vi "通用报警记录浏览.vi"(11 "缓存数据路径":path=path "E:/Program Files (x86)/National Instruments/LabVIEW 2013/data/多点监测缓存数据文件-网络版/2016_10_23 00_23_16 #本机测试端口 #1.60 #1 #PC201410281258_8102.bin") -> ()   [LabVIEW 2017]
uses:
  <vilib>/Utility/miscctls.llb/LVAnnotationListTypeDef.ctl
  <vilib>/event_ctls.llb/eventvkey.ctl
  <vilib>/Utility/NIReport.llb/HTML Report Image Alignment.ctl
  <vilib>/Utility/NIReport.llb/Append Report Text (str wrap).vi
  <vilib>/Utility/NIReport.llb/Append Text Table to Report (wrap).vi
  <vilib>/printing/OpenHTMLReport.llb/Open HTML Report in Browser (Refnum).vi
  <vilib>/Utility/NIReport.llb/NI_report.lvclass
  <vilib>/Utility/NIReport.llb/NI_ReportGenerationCore.lvlib
panel:
  out "标题":string
  out "报警分析":i32(listbox)
  out "探测器信息":i32(listbox)
  out "数值":string
  in  "删除文件":bool
  in  "保存":bool
  out "路径显示":path=path "C:/Users/Administrator/Desktop/35点监测报警信息报表模板 - 副本.doc"
  in  "取消":bool
  in  "生成报表":bool
  in  "结论":string caption="结论（编辑）"
  out "实时曲线":cluster{"X":timestamp[], "Y":dbl[]}[](graph)
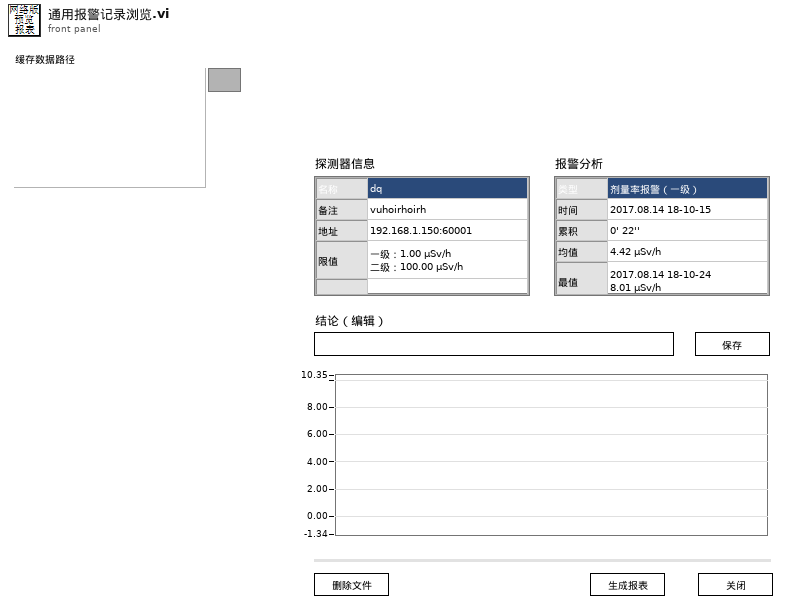
[diagram p1: front panel]
types:
  T1 = typedef "通用报警记录.ctl" = cluster{"探头状态":T2, "探头地址与信息":T3, "缓存绘图数据":T6, "平均值":dbl, "报警时长":cluster{"分":u16, "秒":u16}, "结论":string}
  T2 = typedef "探头状态.ctl" = enum16{"正常", "离线", "禁用", "一级报警", "二级报警", "累积报警"}
  T3 = typedef "探测器信息.ctl" = cluster{"网络地址":string, "名称":string, "备注":string, "累积剂量":dbl, "累积限值":dbl, "硬件剂量率限值":T4, "剂量率限值1":dbl, "剂量率限值2":dbl, "报警方式":T5}
  T4 = typedef "探头剂量率限值选择.ctl" = enum16{"一级限值", "二级限值"}
  T5 = typedef "报警方式选择.ctl" = enum16{"常报警", "自动静音", "手动静音"}
  T6 = typedef "时值缓存压缩模块.lvlib/缓存数据.ctl" = cluster{"时间":timestamp[], "数值":dbl[], "压缩等级数量":i32[], "最大值":cluster{"时间":timestamp, "数值":dbl}, "起始点":cluster{"时间":timestamp, "数值":dbl}, "容量限值":i32, "报警累积":dbl}
  T7 = typedef "LVAnnotationListTypeDef.ctl" = cluster{"Name":string, "Color":u32, "Style":u8, "Point Style":u8, "Name Visible":bool, "Allow Drag":bool, "Annotation Mode":u32, "Plot":i32, "Index":i32, "Position":cluster{"X":dbl, "Y":dbl}, "X Scale":u32, "Y Scale":u32, "Show Arrow":bool, "Lock Name":bool, "Plot Area":i32, "Label Offset":cluster{"X":dbl, "Y":dbl}}[]
  T8 = enum32{"Invalid", "Standard", "Closed", "Hidden", "Minimized", "Maximized"}
  T9 = typedef "eventvkey.ctl" = enum16{"ASCII", "Enter", "Return", "Shift", "Ctrl", "Alt", "Cmd", "Opt", "Caps", "NumLock", "Clear", "Break", "Up", "Down", "Left", "Right", "Insert", "Delete", "Home", "End", "PageUp", "PageDown", "Escape", "Help", "Pause", "ScrollLock", "F1", "F2", "F3", "F4", "F5", "F6", "F7", "F8", "F9", "F10", "F11", "F12", "F13", "F14", "F15", "F16", "F17", "F18", "F19", "F20", "F21", "F22", "F23", "F24", "Play", "VolumeUp", "VolumeDown", "Mute", "Two Byte Char"}
  T10 = enum16{"Standard Report", "HTML", "Word", "Excel"}
  T11 = typedef "NI_ReportGenerationCore.lvlib/HTML Report Image Alignment.ctl" = enum16{"(default)", "LEFT", "RIGHT", "TOP", "TEXTTOP", "MIDDLE", "ABSMIDDLE", "BASELINE", "BOTTOM", "ABSBOTTOM"}
  T12 = cluster{"Name":string, "Color":u32, "Style":u8, "Point Style":u8, "Name Visible":bool, "Allow Drag":bool, "Annotation Mode":u32, "Plot":i32, "Index":i32, "Position":cluster{"X":dbl, "Y":dbl}, "X Scale":u32, "Y Scale":u32, "Show Arrow":bool, "Lock Name":bool, "Plot Area":i32, "Label Offset":cluster{"X":dbl, "Y":dbl}}
  T13 = typedef "LVPoint32TypeDef.ctl" = cluster{"Horizontal":i32, "Vertical":i32}
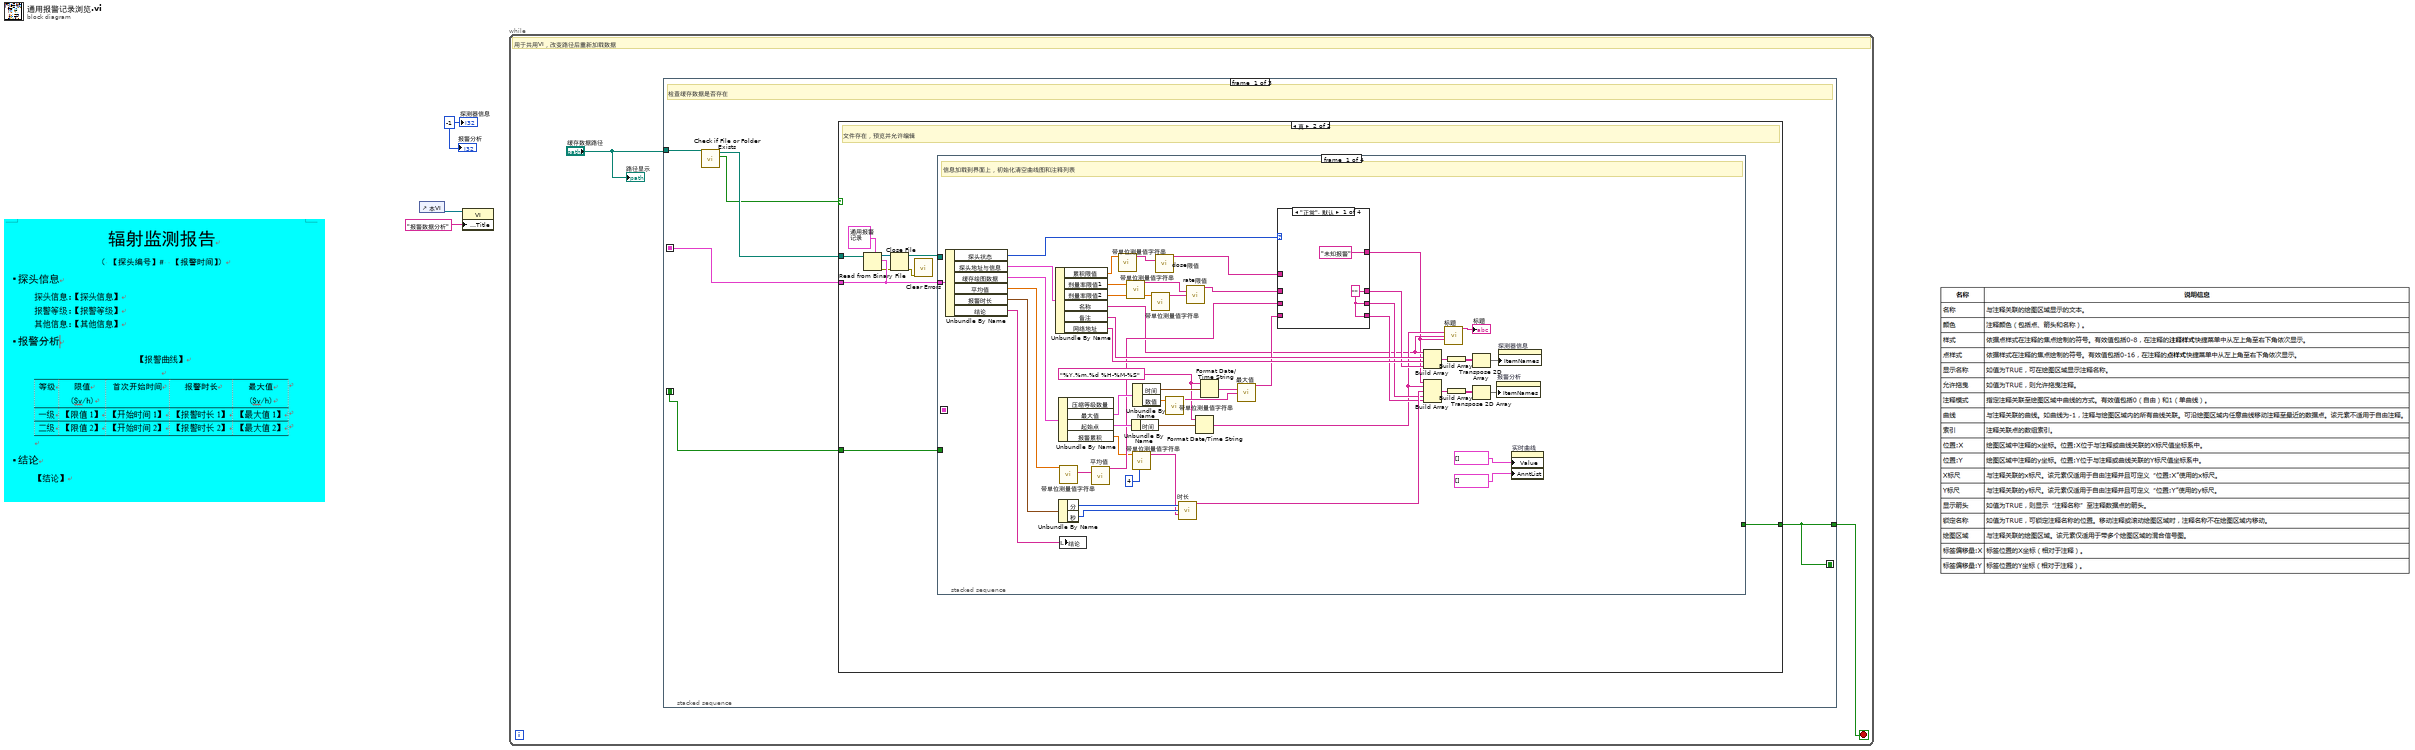
[diagram p0: block diagram]
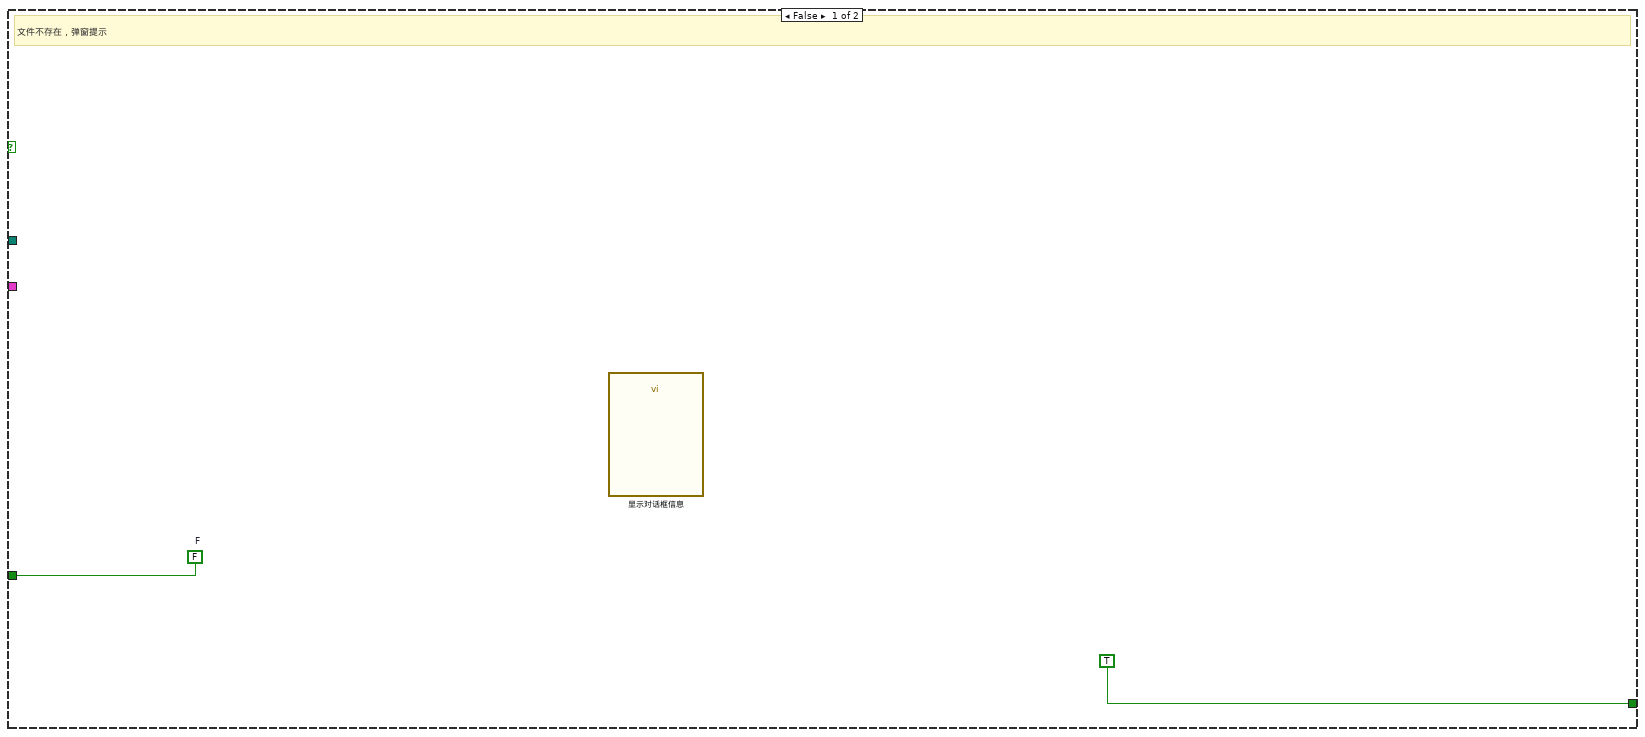
[diagram p2: hidden frame]
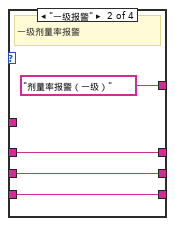
[diagram p3: hidden frame]
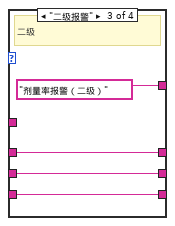
[diagram p4: hidden frame]
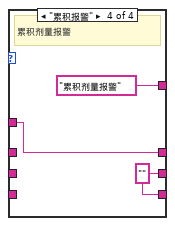
[diagram p5: hidden frame]
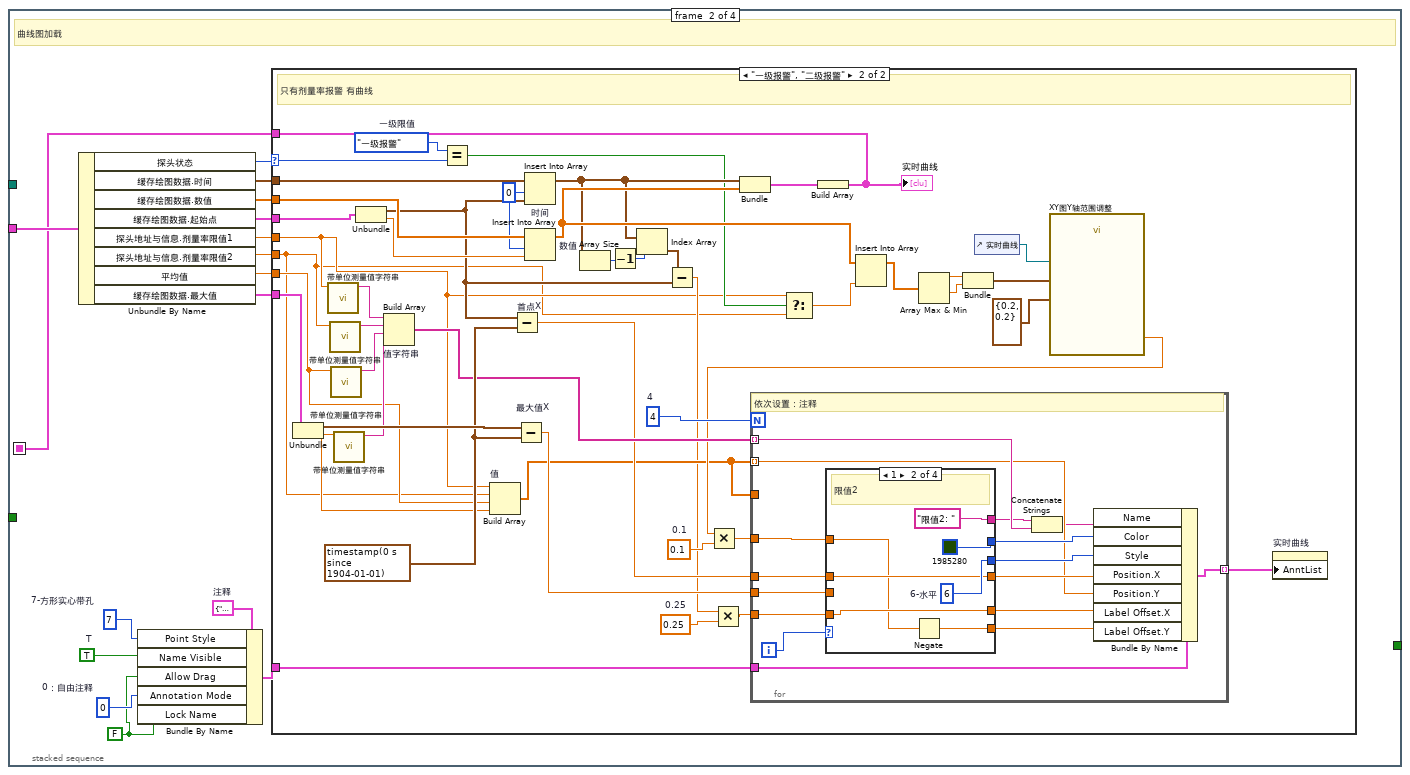
[diagram p6: hidden frame]
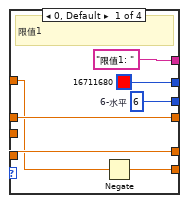
[diagram p8: hidden frame]
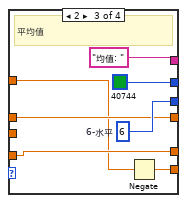
[diagram p9: hidden frame]
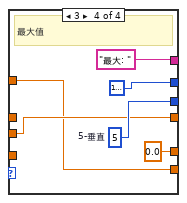
[diagram p10: hidden frame]
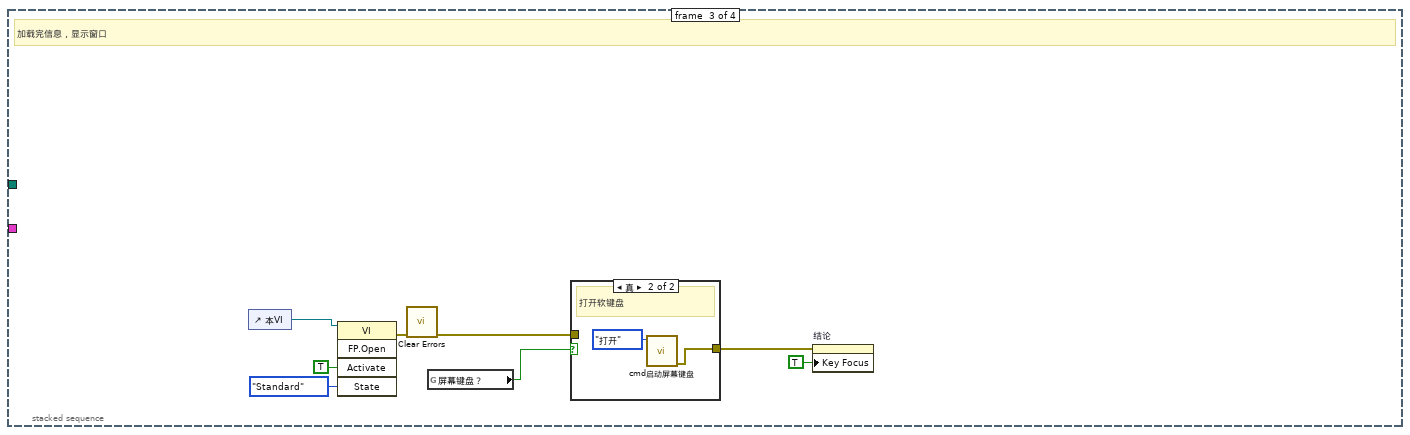
[diagram p11: hidden frame]
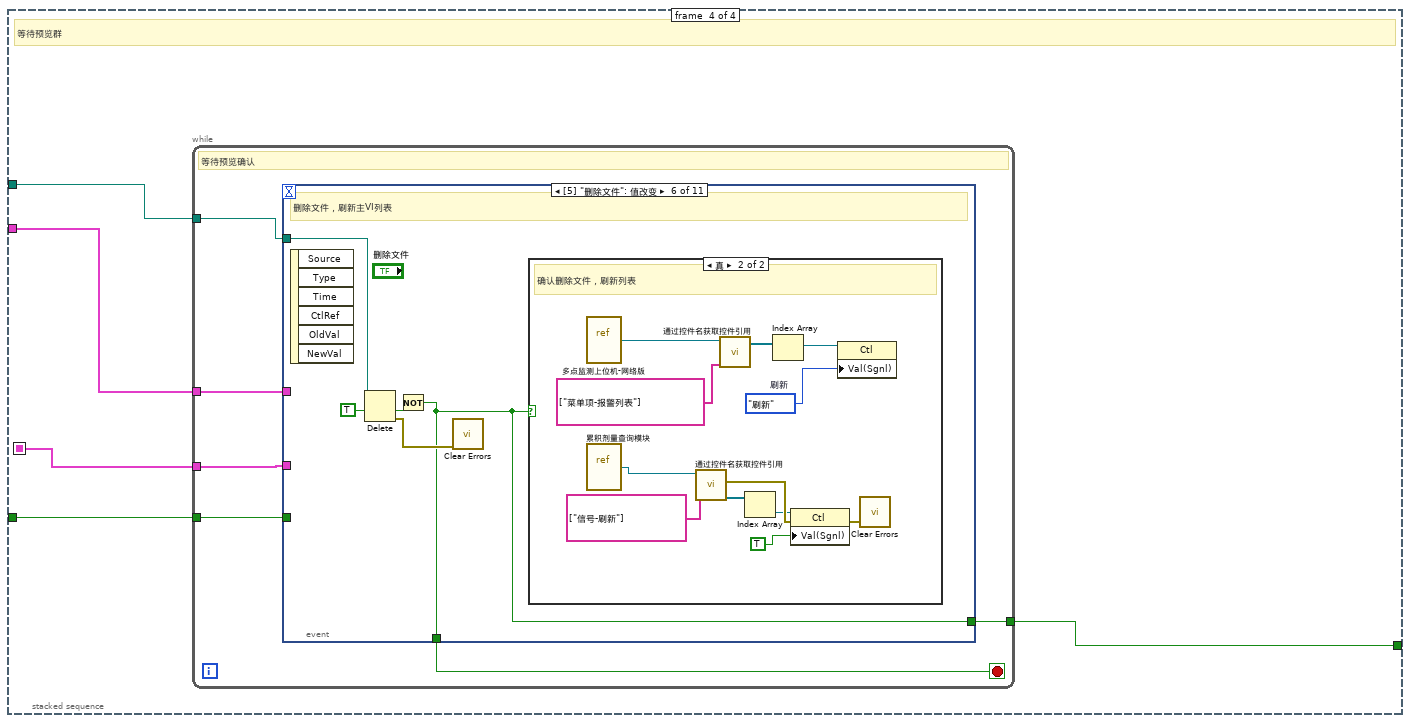
[diagram p13: hidden frame]
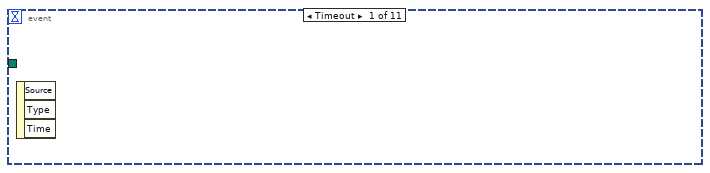
[diagram p14: hidden frame]
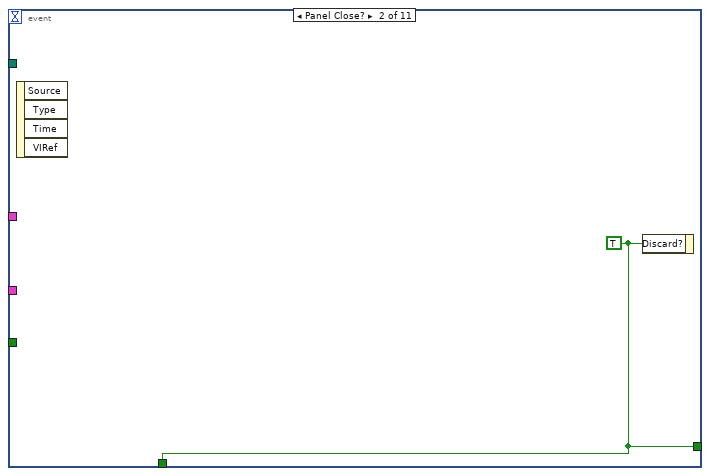
[diagram p15: hidden frame]
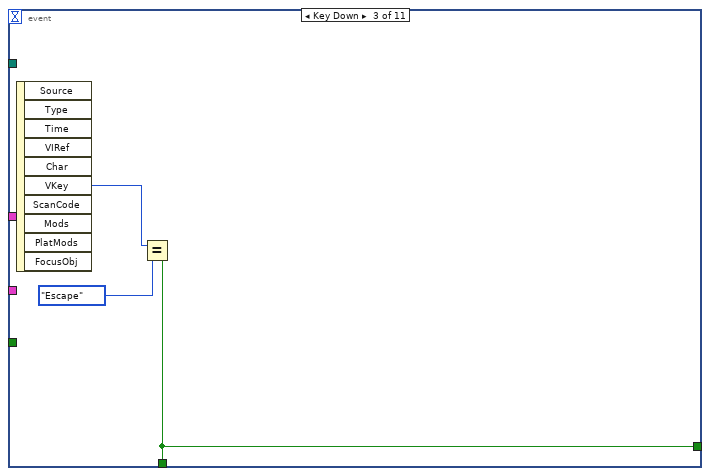
[diagram p16: hidden frame]
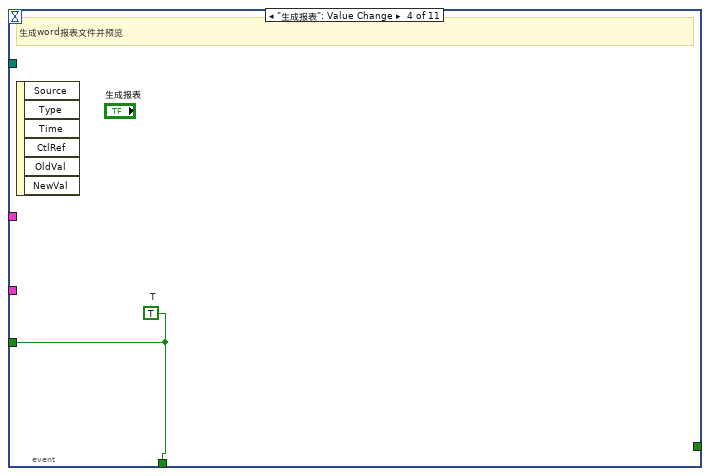
[diagram p17: hidden frame]
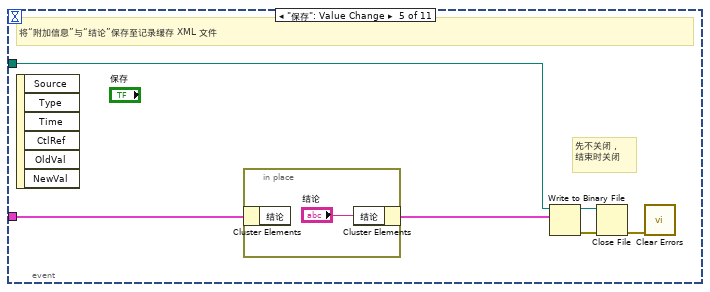
[diagram p18: hidden frame]
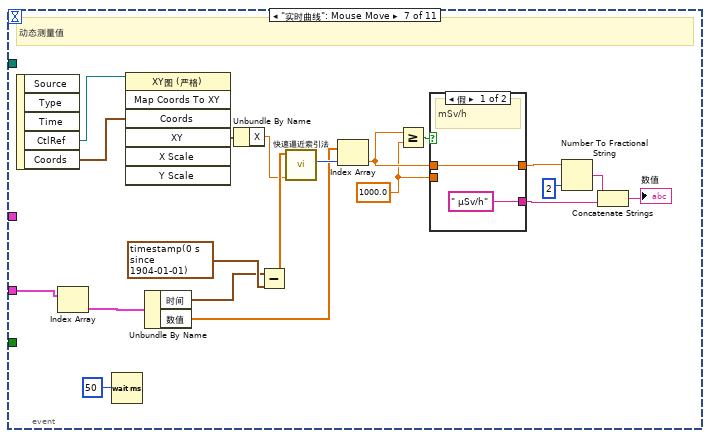
[diagram p20: hidden frame]
diagram:
  w1 = -1 ("探测器信息")
  n1 = control-ref of="本VI"() -> (w2:refnum<vi>)
  n2 = property class="VI"(reference=w2, "Front Panel.Title"="报警数据分析" ("前面板窗口:标题")) -> ()  [unwired: 1 in, 2 out]
  n3 = while {
    stop <- w4 stop-if-true
    # "用于共用VI，改变路径后重新加载数据"
    n4 = stacked-sequence {
      seq-local: [w11 _ _] -> [_ w275 _]
      seq-local: [w10 _ _] -> [_ _ w347]
      seq-local: [w6 _ _] -> [_ w273 _]
      tunnel: "缓存数据路径" -> [w9 w274 _]
      tunnel: [w10 _ _] -> w4
      frame #0 {
        # "检查缓存数据是否存在"
        n5 = call <vilib>:"Check if File or Folder Exists.vi"("path"=w9) -> ("file or folder exists?"=w7:bool, "dup path"=w8:path)  [unwired: 8 in, 1 out]
        n6 = case shown="真" w7 {
          tunnel: [_ w18] -> w6
          tunnel: [w13 w22] -> w11
          tunnel: w8 -> [_ w19]
          tunnel: [TRUE ("T") w21] -> w10
          frame False {
            w13 = FALSE  # F
            # "文件不存在，弹窗提示"
            n7 = call "显示对话框信息"() -> ()  [unwired: 10 in, 2 out]
          }
          frame True {
            # "文件存在，预览并允许编辑"
            n8 = Read from Binary File(5:T1 {"探头状态"=enum."正常", "探头地址与信息"={"网络地址"="", "名称"="", "备注"="", "累积剂量"=0.0, "累积限值"=0.0, "硬件剂量率限值"=enum."一级限值", "剂量率限值1"=0.0, "剂量率限值2"=0.0, "报警方式"=enum."常报警"}, "缓存绘图数据"={"时间"=[], "数值"=[], "压缩等级数量"=[], "最大值"={"时间"=timestamp(0 s since 1904-01-01), "数值"=0.0}, "起始点"={"时间"=timestamp(0 s since 1904-01-01), "数值"=0.0}, "容量限值"=0, "报警累积"=0.0}, "平均值"=0.0, "报警时长"={"分"=0, "秒"=0}, "结论"=""} ("报警记录"), 11:w19) -> (0:w16:errorcluster, 2:w18:T1, 3:w20:refnum<file>)  [unwired: 4 in, 1 out]
            n9 = Close File(refnum=w20, error in=w16) -> (path=w17:path, error out=w15:errorcluster)
            n10 = call <vilib>:"Clear Errors.vi"("error in (no error)"=w15) -> ()  [unwired: 5 in, 2 out]
            n11 = stacked-sequence {
              seq-local: [_ w87 _ _] -> [_ _ _ w201]
              tunnel: w18 -> [w71 w100 _ w204]
              tunnel: [_ _ _ w205] -> w22
              tunnel: w17 -> [_ _ _ w203]
              tunnel: [_ _ _ w202] -> w21
              frame #0 {
                w28 = "%Y.%m.%d %H-%M-%S" ("时间格式字符串(%c)")
                # "信息加载到界面上，初始化清空曲线图和注释列表"
                n12 = Unbundle By Name(w71) -> ("探头状态"=w64:T2, "探头地址与信息"=w69:T3, "缓存绘图数据"=w70:T6, "平均值"=w43:dbl, "报警时长"=w67:cluster{"分":u16, "秒":u16}, "结论"=w68:string)
                n13 = Unbundle By Name(w69) -> ("累积限值"=w61:dbl, "剂量率限值1"=w60:dbl, "剂量率限值2"=w59:dbl, "名称"=w31:string, "备注"=w63:string, "网络地址"=w62:string)
                n14 = Unbundle By Name(w70) -> ("最大值"=w46:cluster{"时间":timestamp, "数值":dbl}, "起始点"=w49:cluster{"时间":timestamp, "数值":dbl}, "报警累积"=w25:dbl)  [unwired: 1 out]
                n15 = Unbundle By Name(w67) -> ("分"=w66:u16, "秒"=w65:u16)
                n16 = local write "结论"(w68) -> ()
                n17 = call "带单位测量值字符串.vi"("测量值"=w43) -> ("结果"=w42:string)  [unwired: 10 in]
                n18 = call "平均值"("平均值"=w42) -> ("Result"=w39:string)  [unwired: 13 in, 1 out]
                n19 = call "带单位测量值字符串.vi"("测量值"=w61) -> ("结果"=w58:string)  [unwired: 10 in]
                n20 = call "带单位测量值字符串.vi"("测量值"=w60) -> ("结果"=w57:string)  [unwired: 10 in]
                n21 = Unbundle By Name(w49) -> ("时间"=w48:timestamp)
                n22 = call "带单位测量值字符串.vi"("精度(2)"=i16 4, "测量值"=w25) -> ("结果"=w24:string)  [unwired: 9 in]
                n23 = Unbundle By Name(w46) -> ("时间"=w45:timestamp, "数值"=w44:dbl)
                n24 = call "带单位测量值字符串.vi"("测量值"=w59) -> ("结果"=w56:string)  [unwired: 10 in]
                n25 = call "dose限值"("限值"=w58) -> ("Result"=w54:string)  [unwired: 13 in, 1 out]
                n26 = call "带单位测量值字符串.vi"("测量值"=w44) -> ("结果"=w40:string)  [unwired: 10 in]
                n27 = call "时长"("分"=w66, "秒"=w65, "累积"=w24) -> ("Result"=w47:string)  [unwired: 11 in, 1 out]
                n28 = call "rate限值"("限值1"=w57, "限值2"=w56) -> ("Result"=w55:string)  [unwired: 12 in, 1 out]
                n29 = Format Date/Time String(time format string (%c)=w28, seconds (now)=w48) -> (date/time string=w32:string)  [unwired: 1 in]
                n30 = Format Date/Time String(time format string (%c)=w28, seconds (now)=w45) -> (date/time string=w41:string)  [unwired: 1 in]
                n31 = call "最大值"("时间"=w41, "最大值"=w40) -> ("Result"=w38:string)  [unwired: 12 in, 1 out]
                n32 = case shown="\"正常\", 默认" w64 {
                  tunnel: ["未知报警" ("字符串") "剂量率报警（一级）" ("字符串") "剂量率报警（二级）" ("字符串") "累积剂量报警" ("字符串")] -> w30
                  tunnel: w55 -> [_ w76 w80 _]
                  tunnel: w54 -> [_ _ _ w83]
                  tunnel: [w72 w76 w80 w83] -> w53
                  tunnel: w39 -> [_ w75 w79 _]
                  tunnel: w38 -> [_ w74 w78 _]
                  tunnel: [w72 w75 w79 w82] -> w37
                  tunnel: [w72 w74 w78 w82] -> w36
                  frame "正常", Default {
                    w72 = "" ("Result")
                  }
                  frame "一级报警" {
                    # "一级剂量率报警"
                  }
                  frame "二级报警" {
                    # "二级"
                  }
                  frame "累积报警" {
                    w82 = "" ("Result")
                    # "累积剂量报警"
                  }
                }
                n33 = Build Array(w31, w63, w62, w53) -> (w52:string[])
                n34 = Build Array(w30, w32, w47, w37, w36) -> (w34:string[])
                n35 = call "标题"("时间"=w32, "名称"=w31, "类型"=w30) -> ("Result"=→"标题":string)  [unwired: 11 in, 1 out]
                n36 = Build Array(w52) -> (w51:string[][])
                n37 = Build Array(w34) -> (w35:string[][])
                n38 = Transpose 2D Array(2D array=w51) -> (transposed array=w50:string[][])
                n39 = Transpose 2D Array(2D array=w35) -> (transposed array=w33:string[][])
                n40 = property on="报警分析" class="MCListbox (严格)"("ItemNames"=w33) -> ()  [unwired: 2 in, 2 out]
                n41 = property on="探测器信息" class="MCListbox (严格)"("ItemNames"=w50) -> ()  [unwired: 2 in, 2 out]
                n42 = property on="实时曲线" class="XY图 (严格)"("Value"=cluster{"X":timestamp[], "Y":dbl[]}[] [] ("实时曲线"), "AnntList"=T7 [] ("注释列表")) -> ()  [unwired: 2 in, 2 out]
              }
              frame #1 {
                w85 = FALSE ("Lock Name")
                w89 = u32 0  # 0：自由注释
                w86 = TRUE  # T
                w90 = 7  # 7-方形实心带孔
                w91 = T12 {"Name"="", "Color"=0, "Style"=0, "Point Style"=0, "Name Visible"=FALSE, "Allow Drag"=FALSE, "Annotation Mode"=0, "Plot"=0, "Index"=0, "Position"={"X"=0.0, "Y"=0.0}, "X Scale"=0, "Y Scale"=0, "Show Arrow"=FALSE, "Lock Name"=FALSE, "Plot Area"=0, "Label Offset"={"X"=0.0, "Y"=0.0}}  # 注释
                # "曲线图加载"
                n43 = Unbundle By Name(w100) -> ("探头状态"=w92:T2, "缓存绘图数据.时间"=w97:timestamp[], "缓存绘图数据.数值"=w98:dbl[], "缓存绘图数据.起始点"=w99:cluster{"时间":timestamp, "数值":dbl}, "探头地址与信息.剂量率限值1"=w96:dbl, "探头地址与信息.剂量率限值2"=w95:dbl, "平均值"=w94:dbl, "缓存绘图数据.最大值"=w93:cluster{"时间":timestamp, "数值":dbl})
                n44 = Bundle By Name(cluster=w91, "Point Style"=w90, "Name Visible"=w86, "Allow Drag"=w85, "Annotation Mode"=w89, "Lock Name"=w85) -> (w88:T12)
                n45 = case shown="\"一级报警\", \"二级报警\"" w92 {
                  selector: w92 -> [_ w106]
                  tunnel: w99 -> [_ w147]
                  tunnel: w98 -> [_ w145]
                  tunnel: w97 -> [_ w143]
                  tunnel: w96 -> [_ w103]
                  tunnel: w95 -> [_ w102]
                  tunnel: w94 -> [_ w132]
                  tunnel: w93 -> [_ w142]
                  tunnel: w88 -> [_ w138]
                  tunnel: [_ w127] -> w87
                  frame "正常", Default {
                  }
                  frame "一级报警", "二级报警" {
                    w105 = 探头状态."一级报警"  # 一级限值
                    w116 = 0.25  # 0.25
                    w118 = 0.1  # 0.1
                    w126 = 0 ("索引")
                    w139 = 4  # 4
                    w140 = timestamp(0 s since 1904-01-01)
                    # "只有剂量率报警 有曲线"
                    n46 = Unbundle(w142) -> ("时间"=w141:timestamp, "数值"=w133:dbl)
                    n47 = call "带单位测量值字符串.vi"("测量值"=w103) -> ("结果"=w137:string)  [unwired: 10 in]
                    n48 = call "带单位测量值字符串.vi"("测量值"=w102) -> ("结果"=w136:string)  [unwired: 10 in]
                    n49 = call "带单位测量值字符串.vi"("测量值"=w132) -> ("结果"=w135:string)  [unwired: 10 in]
                    n50 = call "带单位测量值字符串.vi"("测量值"=w133) -> ("结果"=w134:string)  [unwired: 10 in]
                    n51 = Unbundle(w147) -> ("时间"=w109:timestamp, "数值"=w146:dbl)
                    n52 = Build Array "值字符串"(w137, w136, w135, w134) -> (w131:string[])
                    n53 = Equal?(x=w105, y=w106) -> (x = y?=w104:bool)
                    n54 = Build Array "值"(w103, w102, w132, w133) -> (w114:dbl[])
                    n55 = Subtract "首点X"(x=w109, y=w140) -> (x-y=w130:dbl)
                    n56 = Subtract "最大值X"(x=w141, y=w140) -> (x-y=w129:dbl)
                    n57 = Insert Into Array "时间"(array=w143, index=w126, new element=w109) -> (w112:timestamp[])
                    n58 = Insert Into Array "数值"(array=w145, index=w126, new element=w146) -> (w125:dbl[])
                    n59 = Array Size(array=w112) -> (size(s)=w113:i32)
                    n60 = Decrement(x=w113) -> (x-1=w111:i32)
                    n61 = Index Array(array=w112, index=w111) -> (element=w110:timestamp)
                    n62 = Subtract(x=w110, y=w109) -> (x-y=w108:dbl)
                    n63 = Multiply(x=w108, y=w116) -> (x*y=w115:dbl)
                    n64 = Bundle("时间"=w112, "数值"=w125) -> (w144:cluster{"时间":timestamp[], "数值":dbl[]})  [unwired: 1 in]
                    n65 = Select(t=w103, s=w104, f=w102) -> (s? t:f=w101:dbl)
                    n66 = Build Array(w144) -> (w127:cluster{"时间":timestamp[], "数值":dbl[]}[])
                    "实时曲线" <- w127
                    n67 = Insert Into Array(array=w125, new element=w101) -> (w107:dbl[])  [unwired: 1 in]
                    n68 = Array Max & Min(array=w107) -> (max value=w124:dbl, min value=w123:dbl)  [unwired: 2 out]
                    n69 = Bundle(w124, w123) -> (w122:cluster{dbl, dbl})  [unwired: 1 in]
                    n70 = control-ref of="实时曲线"() -> (w120:refnum<vi>)
                    n71 = call "XY图Y轴范围调整.vi"("留白比例"=cluster{"顶白比例":dbl, "底白比例":dbl} {"顶白比例"=0.2, "底白比例"=0.2}, "最值"=w122, "XY图引用"=w120) -> ("Y轴全长"=w117:dbl)  [unwired: 6 in, 2 out]
                    n72 = Multiply(x=w117, y=w118) -> (x*y=w119:dbl)
                    n73 = for {
                      N: w139 -> [_]
                      tunnel: w138 -> [w162]
                      tunnel: w131 -> [w161] mode=indexing
                      tunnel: w130 -> [w158]
                      tunnel: w129 -> [w157]
                      tunnel: w114 -> [w155] mode=indexing
                      tunnel: w115 -> [w154]
                      tunnel: [w152] -> w128 mode=indexing
                      tunnel: w119 -> [w149]
                      tunnel: w114 -> [_]
                      i -> [w163]
                      # "依次设置：注释"
                      n74 = case shown="1" w163 {
                        tunnel: [u32 16711680 u32 1985280 u32 40744 u32 16777224] -> w160
                        tunnel: [w169 w176 w183 w189] -> w159
                        tunnel: w158 -> [w168 w175 w182 _]
                        tunnel: w157 -> [_ _ _ w186]
                        tunnel: [w168 w175 w182 w186] -> w156
                        tunnel: w154 -> [w167 w174 w181 _]
                        tunnel: [w167 w174 w181 0.0] -> w153
                        tunnel: ["限值1: " "限值2: " "均值: " "最大: "] -> w150
                        tunnel: w149 -> [w165 w172 w179 w185]
                        tunnel: [w164 w171 w178 w185] -> w148
                        frame 0, Default {
                          w169 = u8 6  # 6-水平
                          # "限值1"
                          n75 = Negate(x=w165) -> (-x=w164:dbl)
                        }
                        frame 1 {
                          w176 = u8 6  # 6-水平
                          # "限值2"
                          n76 = Negate(x=w172) -> (-x=w171:dbl)
                        }
                        frame 2 {
                          w183 = u8 6  # 6-水平
                          # "平均值"
                          n77 = Negate(x=w179) -> (-x=w178:dbl)
                        }
                        frame 3 {
                          w189 = u8 5  # 5-垂直
                          # "最大值"
                        }
                      }
                      n78 = Concatenate Strings(w150, w161) -> (w151:string)
                      n79 = Bundle By Name(cluster=w162, "Name"=w151, "Color"=w160, "Style"=w159, "Position.X"=w156, "Position.Y"=w155, "Label Offset.X"=w153, "Label Offset.Y"=w148) -> (w152:T12)
                    }
                    n80 = property on="实时曲线" class="XY图 (严格)"("AnntList"=w128) -> ()  [unwired: 2 in, 2 out]
                  }
                }
              }
              frame #2 {
                # "加载完信息，显示窗口"
                n81 = control-ref of="本VI"() -> (w198:refnum<vi>)
                n82 = invoke class="VI" method="FP.Open"(reference=w198, "Activate"=TRUE ("激活？"), "State"=T8."Standard" ("状态")) -> (error out=w195:errorcluster)  [unwired: 2 in, 4 out]
                n83 = call <vilib>:"Clear Errors.vi"("error in (no error)"=w195) -> ("error out"=w192:errorcluster)  [unwired: 5 in, 1 out]
                n84 = global read "全局变量-35点监测.vi" "屏幕键盘？"() -> (w191:bool)
                n85 = case shown="真" w191 {
                  tunnel: [_ w199] -> w193
                  tunnel: w192 -> [_ _]
                  frame False {
                  }
                  frame True {
                    # "打开软键盘"
                    n86 = call "cmd启动屏幕键盘.vi"("软键盘开关"=enum16{"关闭", "打开"}."打开") -> ("error out"=w199:errorcluster)  [unwired: 9 in, 1 out]
                  }
                }
                n87 = property on="结论" class="Str"(error in=w193, "Key Focus"=TRUE ("键选中")) -> ()  [unwired: 1 in, 2 out]
              }
              frame #3 {
                # "等待预览群"
                n88 = while {
                  tunnel: [w210] -> w205
                  tunnel: w204 -> [w209]
                  tunnel: w203 -> [w208]
                  tunnel: [w207] -> w202
                  tunnel: w201 -> [w206]
                  stop <- w211 stop-if-true
                  # "等待预览确认"
                  n89 = event shown="[5] \"删除文件\": 值改变" {
                    selector: _ -> [_ _ _ _ _ _ _ _ _ _ _]
                    dyn-events: _ -> [_ _ _ _ _ _ _ _ _ _ _]
                    timeout: _ -> [_ _ _ _ _ _ _ _ _ _ _]
                    tunnel: [_ w212 w213 w216 _ w224 _ _ _ TRUE ("T") w271] -> w211
                    tunnel: [_ _ _ w216 _ _ _ _ _ _ w272] -> w210
                    tunnel: w209 -> [_ _ _ _ w222 _ _ _ _ _ _]
                    tunnel: w208 -> [_ _ _ _ w221 w227 _ _ _ _ _]
                    tunnel: [_ w212 w213 _ _ w224 _ _ _ FALSE ("T") w271] -> w207
                    tunnel: w206 -> [_ _ _ _ _ _ w241 _ _ _ _]
                    event Timeout {
                      n90 = event-data() -> ()  [unwired: 1 in, 3 out]
                    }
                    event Panel Close? {
                      w212 = TRUE ("放弃？")
                      n91 = event-data() -> ()  [unwired: 1 in, 4 out]
                      n92 = event-data("Discard?"=w212) -> ()  [unwired: 1 in, 1 out]
                    }
                    event Key Down {
                      n93 = event-data() -> ("VKey"=w215:T9)  [unwired: 1 in, 9 out]
                      n94 = Equal?(x=w215, y=eventvkey."Escape") -> (x = y?=w213:bool)
                    }
                    event "生成报表": Value Change {
                      w216 = TRUE  # T
                      # "生成word报表文件并预览"
                      n95 = event-data() -> ()  [unwired: 1 in, 6 out]
                    }
                    event "保存": Value Change {
                      # "先不关闭，\n结束时关闭"
                      # "将“附加信息”与“结论”保存至记录缓存 XML 文件"
                      n96 = event-data() -> ()  [unwired: 1 in, 6 out]
                      n97 = in-place {
                        n98 = in-place-cluster #1(w222) -> ()  [unwired: 1 out]
                        n99 = in-place-cluster #1("结论"="结论") -> (w220:T1)
                      }
                      n100 = Write to Binary File(file (use dialog)=w221, data=w220) -> (refnum out=w217:refnum<file>, error out=w219:errorcluster)  [unwired: 4 in, 1 out]
                      n101 = Close File(refnum=w217, error in=w219) -> (error out=w218:errorcluster)  [unwired: 1 out]
                      n102 = call <vilib>:"Clear Errors.vi"("error in (no error)"=w218) -> ()  [unwired: 5 in, 2 out]
                    }
                    event "删除文件": Value Change {
                      # "删除文件，刷新主VI列表"
                      n103 = event-data() -> ()  [unwired: 1 in, 6 out]
                      n104 = Delete(path (use dialog)=w227, confirm (F)=TRUE ("确认(F)")) -> (cancelled=w225:bool, error out=w228:errorcluster)  [unwired: 3 in, 1 out]
                      n105 = Not(x=w225) -> (.not. x?=w224:bool)
                      n106 = call <vilib>:"Clear Errors.vi"("error in (no error)"=w228) -> ()  [unwired: 5 in, 2 out]
                      n107 = case shown="真" w224 {
                        frame False {
                          # "取消删除"
                        }
                        frame True {
                          w236 = enum16{"刷新", "预览并生成报表", "删除记录", "复制选中项至剪贴板"}."刷新"  # 刷新
                          # "确认删除文件，刷新列表"
                          n108 = vi-ref "多点监测上位机-网络版.vi"() -> (w240:refnum<vi>)
                          n109 = vi-ref "累积剂量查询模块.vi"() -> (w230:refnum<vi>)
                          n110 = call "通过控件名获取控件引用.vi"("控件名数组"=string[] ["信号-刷新"], "VI引用"=w230) -> ("控件引用输出"=w231:refnum<vi>[], "错误输出"=w234:errorcluster)  [unwired: 7 in, 1 out]
                          n111 = call "通过控件名获取控件引用.vi"("控件名数组"=string[] ["菜单项-报警列表"], "VI引用"=w240) -> ("控件引用输出"=w238:refnum<vi>[])  [unwired: 7 in, 2 out]
                          n112 = Index Array(array=w231) -> (element=w232:refnum<vi>)  [unwired: 1 in]
                          n113 = Index Array(array=w238) -> (element=w237:refnum<vi>)  [unwired: 1 in]
                          n114 = property class="Ctl"(reference=w232, error in=w234, "Val(Sgnl)"=TRUE) -> (error out=w235:errorcluster)  [unwired: 1 out]
                          n115 = property class="Ctl"(reference=w237, "Val(Sgnl)"=w236) -> ()  [unwired: 1 in, 2 out]
                          n116 = call <vilib>:"Clear Errors.vi"("error in (no error)"=w235) -> ()  [unwired: 5 in, 2 out]
                        }
                      }
                    }
                    event "实时曲线": Mouse Move {
                      w248 = 1000.0 ("y")
                      # "动态测量值"
                      n117 = event-data() -> ("CtlRef"=w243:refnum<vi>, "Coords"=w244:T13)  [unwired: 1 in, 3 out]
                      n118 = Index Array(array=w241) -> (element=w242:cluster{"时间":timestamp[], "数值":dbl[]})  [unwired: 1 in]
                      n119 = Wait (ms)(milliseconds to wait=u32 50 ("等待时间（毫秒）")) -> ()  [unwired: 1 out]
                      n120 = invoke on="调用节点" class="XY图 (严格)" method="Map Coords To XY"(reference=w243, "Coords"=w244) -> ("XY"=w246:cluster{"X":dbl, "Y":dbl})  [unwired: 5 in, 6 out]
                      n121 = Unbundle By Name(w242) -> ("时间"=w255:timestamp[], "数值"=w258:dbl[])
                      n122 = Unbundle By Name(w246) -> ("X"=w254:dbl)
                      n123 = Subtract(x=w255, y=timestamp(0 s since 1904-01-01)) -> (x-y=w257:dbl[])
                      n124 = call "快速逼近索引法.vi"("数值"=w254, "数组"=w257) -> ("最近索引"=w259:i32)  [unwired: 9 in]
                      n125 = Index Array(array=w258, index=w259) -> (element=w260:dbl)
                      n126 = Greater Or Equal?(x=w260, y=w248) -> (x >= y?=w247:bool)
                      n127 = case shown="假" w247 {
                        tunnel: w260 -> [w262 w266]
                        tunnel: w248 -> [_ w265]
                        tunnel: [w262 w264] -> w250
                        tunnel: [" μSv/h" " mSv/h"] -> w252
                        frame False {
                          # "mSv/h"
                        }
                        frame True {
                          # "uSv/h"
                          n128 = Divide(x=w266, y=w265) -> (x/y=w264:dbl)
                        }
                      }
                      n129 = Number To Fractional String(number=w250, precision (6)=i16 2 ("精度(6)")) -> (F-format string=w251:string)  [unwired: 2 in]
                      n130 = Concatenate Strings(w251, w252) -> (→"数值":string)
                    }
                    event "实时曲线": Mouse Enter {
                      # "显示 动态测量值"
                      n131 = event-data() -> ()  [unwired: 1 in, 4 out]
                      n132 = property on="数值" class="Str"("Visible"=TRUE ("可见")) -> ()  [unwired: 2 in, 2 out]
                    }
                    event "实时曲线": Mouse Leave {
                      # "隐藏 动态测量值"
                      n133 = event-data() -> ()  [unwired: 1 in, 4 out]
                      n134 = property on="数值" class="Str"("Visible"=FALSE ("可见")) -> ()  [unwired: 2 in, 2 out]
                    }
                    event "缓存数据路径": Value Change {
                      # "重新加载与分析数据，结束当前循环"
                      n135 = event-data() -> ()  [unwired: 1 in, 6 out]
                    }
                    event "取消": Value Change {
                      w272 = FALSE  # F
                      w271 = TRUE  # T
                      # "取消生成"
                      n136 = event-data() -> ()  [unwired: 1 in, 6 out]
                    }
                  }
                }
              }
            }
          }
        }
      }
      frame #1 {
        # "是否生成报表"
        n137 = case shown="真" w275 {
          tunnel: w274 -> [_ _]
          tunnel: w273 -> [_ w337]
          frame False {
            # "缓存数据不存在，或点击“取消”"
          }
          frame True {
            w290 = 1.75
            w324 = enum16{"H1", "H2", "H3", "H4", "H5", "H6", "H7"}."H3"  # H1
            w315 = FALSE  # F
            w302 = TRUE  # T
            w332 = TRUE  # T
            w298 = FALSE  # F
            # "缓存数据存在，并点击“生成报表”，生成 HTML 报表"
            n138 = Unbundle By Name(w337) -> ("探头状态"=w310:T2)
            n139 = local read "标题"() -> (w326:string)
            n140 = call <vilib>:"New Report.vi"("report type"=T10."HTML") -> ("report out"=w328:refnum<class "NI_report.lvclass">, "error out"=w327:errorcluster)  [unwired: 13 in]
            n141 = call-dynamic "Set Report Header Text.vi"("report in"=w328, "center header text"=w326, "error in (no error)"=w327, "HTML header size"=w324, "header placement"=enum16{"Top of Document", "Append to Body"}."Append to Body") -> ("report out"=w320:refnum<class "NI_report.lvclass">, "error out"=w319:errorcluster)  [unwired: 9 in]
            n142 = property on="探测器信息" class="MCListbox (严格)"() -> ("RowHdrs[]"=w314:string[], "ItemNames"=w313:string[][])  [unwired: 2 in, 2 out]
            n143 = call-poly <vilib>:"Append Report Text.vi"("report in"=w320, "text"="\n一、探测器信息\n", "append on new line? (F)"=w302, "error in (no error)"=w319) -> ("report out"=w282:refnum<class "NI_report.lvclass">, "error out"=w283:errorcluster)  [unwired: 8 in, 2 out]
            n144 = call-dynamic "New Report Line.vi"("report in"=w282, "error in (no error)"=w283) -> ("report out"=w281:refnum<class "NI_report.lvclass">, "error out"=w280:errorcluster)  [unwired: 12 in]
            n145 = call-poly <vilib>:"Append Table to Report.vi"("report in"=w281, "column width (1)"=w290, "row headers"=w314, "text data"=w313, "error in (no error)"=w280, "show grid lines (YES)"=w315) -> ("report out"=w284:refnum<class "NI_report.lvclass">, "error out"=w285:errorcluster)  [unwired: 6 in, 2 out]
            n146 = property on="报警分析" class="MCListbox (严格)"() -> ("RowHdrs[]"=w312:string[], "ItemNames"=w311:string[][])  [unwired: 2 in, 2 out]
            n147 = call-poly <vilib>:"Append Report Text.vi"("report in"=w284, "text"="二、报警分析\n", "append on new line? (F)"=w302, "error in (no error)"=w285) -> ("report out"=w289:refnum<class "NI_report.lvclass">, "error out"=w287:errorcluster)  [unwired: 8 in, 2 out]
            n148 = call-dynamic "New Report Line.vi"("report in"=w289, "error in (no error)"=w287) -> ("report out"=w288:refnum<class "NI_report.lvclass">, "error out"=w286:errorcluster)  [unwired: 12 in]
            n149 = call-poly <vilib>:"Append Table to Report.vi"("report in"=w288, "column width (1)"=w290, "row headers"=w312, "text data"=w311, "error in (no error)"=w286, "show grid lines (YES)"=w315) -> ("report out"=w278:refnum<class "NI_report.lvclass">, "error out"=w279:errorcluster)  [unwired: 6 in, 2 out]
            n150 = call-dynamic "New Report Line.vi"("report in"=w278, "error in (no error)"=w279) -> ("report out"=w277:refnum<class "NI_report.lvclass">, "error out"=w276:errorcluster)  [unwired: 12 in]
            n151 = case shown="\"一级报警\", \"二级报警\"" w310 {
              tunnel: w277 -> [w339 w346]
              tunnel: w276 -> [w338 w345]
              tunnel: [w338 w341] -> w309
              tunnel: [w339 w340] -> w308
              frame "禁用", Default {
                # "累积剂量报警没有曲线图"
              }
              frame "一级报警", "二级报警" {
                # "剂量率报警有曲线图"
                n152 = control-ref of="实时曲线"() -> (w344:refnum<vi>)
                n153 = call-dynamic "Append Control Image to Report.vi"("report in"=w346, "alignment (default)"=HTML_Report_Image_Alignment."MIDDLE", "image file type (.jpg)"=enum16{".jpg", ".png"}.".png", "ctrl reference"=w344, "error in (no error)"=w345) -> ("report out"=w340:refnum<class "NI_report.lvclass">, "error out"=w341:errorcluster)  [unwired: 7 in, 2 out]
              }
            }
            n154 = call "路径查找创建-报警记录清单-网络版.vi"() -> ("报表文件夹"=w331:path)  [unwired: 2 in, 13 out]
            n155 = call-poly <vilib>:"Append Report Text.vi"("report in"=w308, "text"="\n三、结论\n", "append on new line? (F)"=w302, "error in (no error)"=w309) -> ("report out"=w317:refnum<class "NI_report.lvclass">, "error out"=w316:errorcluster)  [unwired: 8 in, 2 out]
            n156 = local read "结论"() -> (w318:string)
            n157 = call-poly <vilib>:"Append Report Text.vi"("report in"=w317, "text"=w318, "append on new line? (F)"=w302, "error in (no error)"=w316) -> ("report out"=w305:refnum<class "NI_report.lvclass">, "error out"=w306:errorcluster)  [unwired: 8 in, 2 out]
            n158 = call-dynamic "New Report Line.vi"("report in"=w305, "number of lines (1)"=2, "error in (no error)"=w306) -> ("report out"=w304:refnum<class "NI_report.lvclass">, "error out"=w303:errorcluster)  [unwired: 11 in]
            n159 = Concatenate Strings(w326, ".html" ("字符串")) -> (w296:string)
            n160 = call-dynamic "Append Horizontal Line to Report.vi"("report in"=w304, "error in (no error)"=w303) -> ("report out"=w301:refnum<class "NI_report.lvclass">, "error out"=w299:errorcluster)  [unwired: 12 in]
            n161 = call-poly <vilib>:"Append Report Text.vi"("report in"=w301, "text"="验证人：\n\n日期：\n", "append on new line? (F)"=w302, "error in (no error)"=w299) -> ("report out"=w295:refnum<class "NI_report.lvclass">, "error out"=w294:errorcluster)  [unwired: 8 in, 2 out]
            n162 = Build Path(base path=w331, name or relative path=w296) -> (appended path=w329:path)
            n163 = call-dynamic "New Report Line.vi"("report in"=w295, "error in (no error)"=w294) -> ("report out"=w292:refnum<class "NI_report.lvclass">, "error out"=w293:errorcluster)  [unwired: 12 in]
            n164 = call-poly <vilib>:"Open HTML Report in Browser.vi"("report in"=w292, "error in (no error)"=w293) -> ("report out"=w335:refnum<class "NI_report.lvclass">, "error out"=w297:errorcluster)  [unwired: 11 in, 1 out]
            n165 = call-dynamic "Save Report to File.vi"("report in"=w335, "report file path"=w329, "error in (no error)"=w297) -> ("report out"=w334:refnum<class "NI_report.lvclass">, "error out"=w333:errorcluster)  [unwired: 11 in]
            n166 = call-dynamic "Dispose Report.vi"("report in"=w334, "wait until printing completed? (T)"=w298, "save changes? (F)"=w332, "error in (no error)"=w333) -> ("error out"=w291:errorcluster)  [unwired: 11 in]
            n167 = call <vilib>:"Simple Error Handler.vi"("error in (no error)"=w291) -> ()  [unwired: 4 in, 5 out]
          }
        }
      }
      frame #2 {
        # "退出关闭本VI"
        n168 = case shown="真" w347 {
          frame False {
          }
          frame True {
            # "结束程序？"
            n169 = control-ref of="本VI"() -> (w353:refnum<vi>)
            n170 = call "cmd启动屏幕键盘.vi"("软键盘开关"=enum16{"关闭", "打开"}."关闭") -> ("error out"=w348:errorcluster)  [unwired: 9 in, 1 out]
            n171 = invoke class="VI" method="FP.Close"(reference=w353, error in=w348) -> (reference out=w352:refnum<vi>, error out=w351:errorcluster)  [unwired: 1 in, 1 out]
            n172 = invoke class="VI" method="Abort VI"(reference=w352, error in=w351) -> (error out=w350:errorcluster)  [unwired: 1 in, 2 out]
            n173 = call <vilib>:"Clear Errors.vi"("error in (no error)"=w350) -> ()  [unwired: 5 in, 2 out]
          }
        }
      }
    }
    "路径显示" <- "缓存数据路径"
  }
  "探测器信息" <- w1
  "报警分析" <- w1
